vi "Java_killer.vi"(8 "error in (no error)":errorcluster) -> (0 "error out":errorcluster)   [LabVIEW 2019]
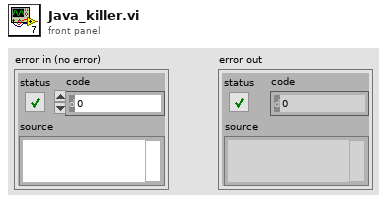
[diagram p1: front panel]
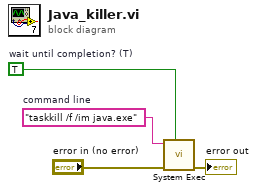
[diagram p0: block diagram]
diagram:
  w4 = TRUE  # wait until completion? (T)
  w3 = "taskkill /f /im java.exe"  # command line
  n1 = call <vilib>:"System Exec.vi"("wait until completion? (T)"=w4, "error in (no error)"="error in (no error)", "command line"=w3) -> ("error out"=→"error out":errorcluster)  [unwired: 5 in, 3 out]
